vi "VI Tree - file.vi"() -> ()   [LabVIEW 2009]
uses:
  Strip Path/Strip Path - Traditional.vi
  Build Path/Build Path - Traditional.vi
  File Exists/File Exists - Scalar.vi
  Strip Path Extension/Strip Path Extension - Path.vi
  Valid Path/Valid Path - Traditional.vi
  Convert File Extension/Convert File Extension (Path).vi
  Compare Two Paths/Compare Two Paths - Scalar.vi
panel:
  in  "Case Constant\n(See Context Help)":bool
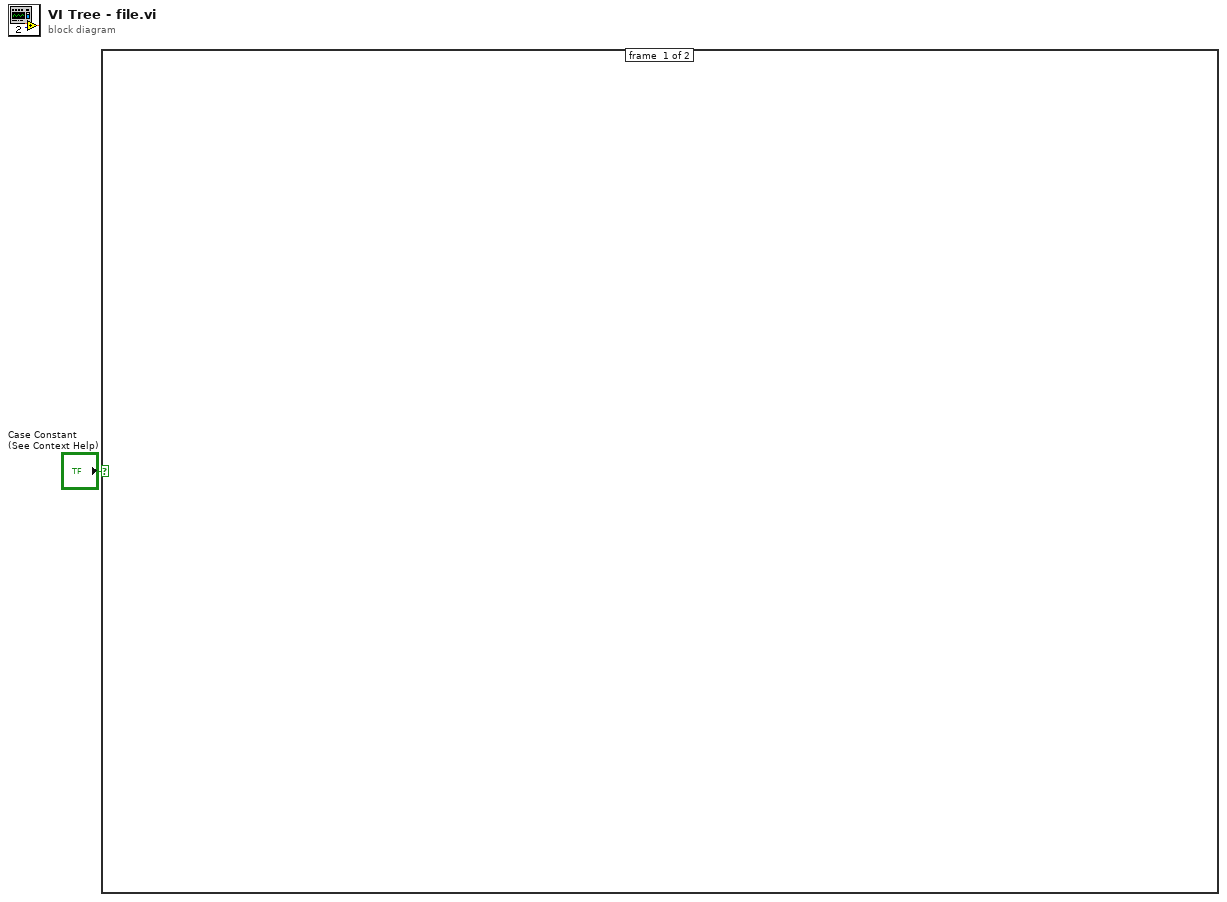
[diagram p0: block diagram]
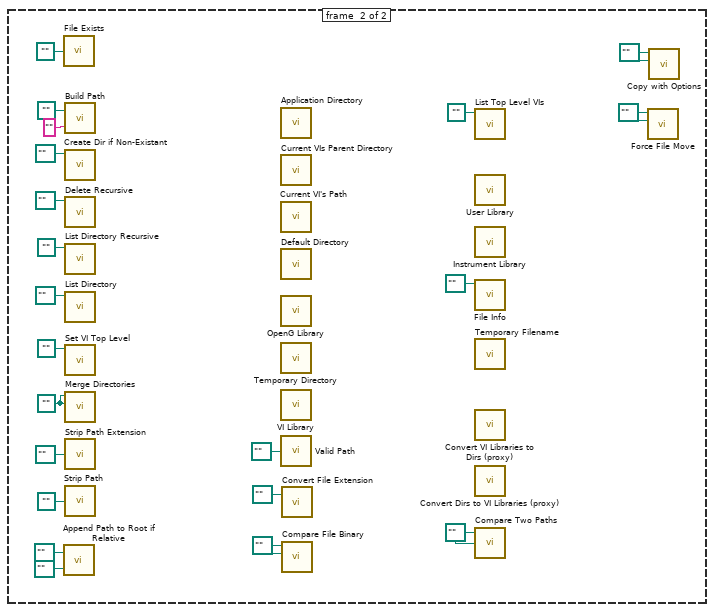
[diagram p2: hidden frame]
diagram:
  n1 = case shown="True" "Case Constant\n(See Context Help)" {
    frame #0 {
    }
    frame #1 {
      w2 = path "" ("target")
      w3 = path "" ("source path")
      w4 = path "" ("path1")
      w6 = path "" ("original file")
      w19 = path "" ("target directory path")
      n2 = call-poly "File Exists.vi"("file path"=path "") -> ()  [unwired: 6 in, 2 out]
      n3 = call "Append Path to Root if Relative.vi"("Absolute or Relative Path"=path "", "Root Path"=path "") -> ()  [unwired: 1 out]
      n4 = call-poly "Build Path.vi"("name or relative path"="", "base path"=path "") -> ()  [unwired: 1 out]
      n5 = call "Create Dir if Non-Existant.vi"("Directory Path"=path "") -> ()  [unwired: 8 in, 3 out]
      n6 = call "Delete Recursive.vi"("Path"=path "") -> ()  [unwired: 9 in, 2 out]
      n7 = call "List Directory Recursive.vi"("Path"=path "") -> ()  [unwired: 7 in, 4 out]
      n8 = call "List Directory.vi"("directory path"=path "") -> ()  [unwired: 3 in, 4 out]
      n9 = call "Set VI Top Level.vi"("VI Path"=path "") -> ()  [unwired: 9 in, 2 out]
      n10 = call "Merge Directories.vi"("target directory path"=w19, "source directory path"=w19) -> ()  [unwired: 8 in, 2 out]
      n11 = call-poly "Strip Path Extension.vi"("path"=path "") -> ()  [unwired: 2 out]
      n12 = call-poly "Strip Path.vi"("path"=path "") -> ()  [unwired: 2 out]
      n13 = call "Application Directory.vi"() -> ()  [unwired: 1 in, 1 out]
      n14 = call "Current VIs Parent Directory.vi"() -> ()  [unwired: 5 in, 1 out]
      n15 = call "Current VI's Path.vi"() -> ()  [unwired: 1 in, 1 out]
      n16 = call "Default Directory.vi"() -> ()  [unwired: 1 in, 1 out]
      n17 = call "OpenG Library.vi"() -> ()  [unwired: 1 in, 1 out]
      n18 = call "Temporary Directory.vi"() -> ()  [unwired: 1 in, 1 out]
      n19 = call "VI Library.vi"() -> ()  [unwired: 1 in, 1 out]
      n20 = call-poly "Valid Path.vi"("path"=path "") -> ()  [unwired: 1 out]
      n21 = call-poly "Convert File Extension.vi"("file name"=path "") -> ()  [unwired: 1 in, 2 out]
      n22 = call "Compare File Binary.vi"("copy file"=w6, "original file"=w6) -> ()  [unwired: 4 in, 2 out]
      n23 = call "List Top Level VIs.vi"("LLB Path"=path "") -> ()  [unwired: 8 in, 3 out]
      n24 = call "User Library.vi"() -> ()  [unwired: 1 in, 1 out]
      n25 = call "Instrument Library.vi"() -> ()  [unwired: 1 in, 1 out]
      n26 = call "File Info.vi"("file"=path "") -> ()  [unwired: 5 in, 3 out]
      n27 = call "Temporary Filename.vi"() -> ()  [unwired: 6 in, 2 out]
      n28 = call "Convert VI Libraries to Dirs (proxy).vi"() -> ()  [unwired: 8 in, 4 out]
      n29 = call "Convert Dirs to VI Libraries (proxy).vi"() -> ()  [unwired: 11 in, 1 out]
      n30 = call-poly "Compare Two Paths.vi"("path2"=w4, "path1"=w4) -> ()  [unwired: 1 in, 3 out]
      n31 = call "Force File Move.vi"("source"=w2, "target"=w2) -> ()  [unwired: 4 in, 2 out]
      n32 = call "Copy with Options.vi"("target path"=w3, "source path"=w3) -> ()  [unwired: 8 in, 2 out]
    }
  }
